vi "Display Screen.vi"(7 "Screen (Channels A & B)":u16(ring)=2 items=["Channel A", "Channel B", "Channels A & B", "User"], 8 "error in (no error)":errorcluster, 10 "Node In":string, 11 "VISA resource name":refnum<visa-resource-name>) -> (0 "error out":errorcluster, 2 "Node Out":string, 3 "VISA resource name out":refnum<visa-resource-name>, 4 "Command String":string)   [LabVIEW 2018, in "Keithley 2600 Series.lvlib"]
doc: "Changes the screen displayed on the front pannel of the 26xx.\n\n<b>Functions and Attributes Used</b>\ndisplay.screen"
uses:
  Keithley 2600 Series.lvlib
  Private/GlobalVariables.vi
panel:
  # "(c) 2008 Keithley Instruments, Inc.  ALL RIGHTS RESERVED."
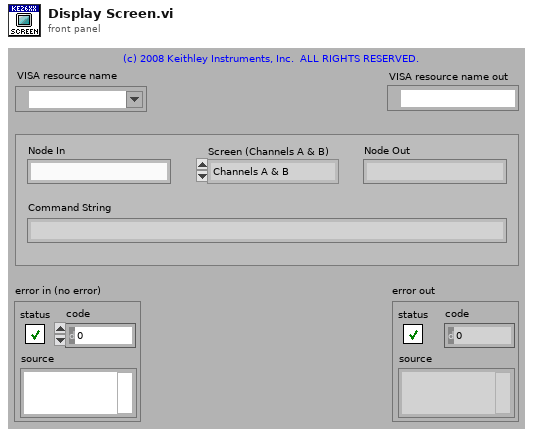
[diagram p1: front panel]
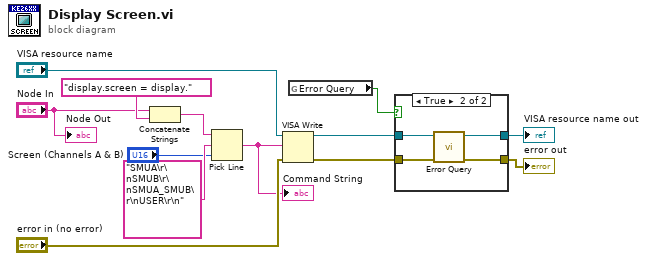
[diagram p0: block diagram]
diagram:
  n1 = Concatenate Strings("Node In", "display.screen = display." ("command")) -> (w11:string)
  n2 = Pick Line(string ("")=w11, multi-line string="SMUA\r\nSMUB\r\nSMUA_SMUB\r\nUSER\r\n" ("options"), line index="Screen (Channels A & B)") -> (output string=w6:string)
  "Command String" <- w6
  n3 = VISA Write(VISA resource name="VISA resource name", write buffer=w6, error in (no error)="error in (no error)") -> (VISA resource name out=w4:refnum<visa-resource-name>, error out=w3:errorcluster)  [unwired: 1 out]
  n4 = global read "GlobalVariables.vi" "Error Query"() -> (w5:bool)
  n5 = case shown="True" w5 {
    tunnel: w4 -> [w15 w19]
    tunnel: w3 -> [w14 w18]
    tunnel: [w15 w17] -> w2
    tunnel: [w14 w16] -> w1
    frame False {
    }
    frame True {
      n6 = call "Error Query.vi"("error in (no error)"=w18, "VISA resource name"=w19) -> ("error out"=w16:errorcluster, "VISA resource name out"=w17:refnum<visa-resource-name>)  [unwired: 8 out]
    }
  }
  "VISA resource name out" <- w2
  "error out" <- w1
  "Node Out" <- "Node In"
